vi "Teleop.vi"(10 "Match Info":T1={"Autonomous Elapsed Seconds"=0.0, "TeleOp Elapsed Seconds"=0.0, "Disabled Elapsed Seconds"=0.0, "Visited Autonomous"=FALSE, "Visited TeleOp"=FALSE, "Visited Disabled"=FALSE, "Autonomous Settings"={"Autonomous Style"=enum."Independent", "VI Refnum"=refnum}}, 11 "Call Context":T2) -> ()   [LabVIEW 2013]
doc: "This VI is called for each TeleOp packet received from the DS where the robot is not disabled. It is often used to read from the joysticks and update I/O or to update setpoints for timed control loops. It should complete and return within 20 milliseconds or it may miss DS packets."
uses:
  <vilib>/Rock Robotics/WPI/DriverStation/WPI_DriverStationDerivedRobotMode.ctl
  <vilib>/Rock Robotics/WPI/DriverStation/WPI_DriverStationMatch Info.ctl
  Robot Global Data.vi
  Gyro/Gyro Global.vi
  <vilib>/Rock Robotics/WPI/Joystick/WPI_JoystickGetSetRefNum.vi
panel:
  out "back":dbl
  out "front":dbl
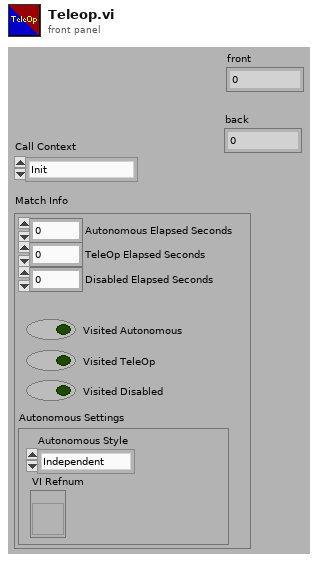
[diagram p1: front panel]
types:
  T1 = typedef "WPI_DriverStationMatch Info.ctl" = cluster{"Autonomous Elapsed Seconds":dbl, "TeleOp Elapsed Seconds":dbl, "Disabled Elapsed Seconds":dbl, "Visited Autonomous":bool, "Visited TeleOp":bool, "Visited Disabled":bool, "Autonomous Settings":cluster{"Autonomous Style":enum16{"Iterative", "Independent"}, "VI Refnum":refnum<vi>}}
  T2 = typedef "WPI_DriverStationDerivedRobotMode.ctl" = enum16{"Init", "Execute", "Stop"}
  T3 = typedef "WPI_JoystickDevRef.ctl" = cluster{"Device":T4}
  T4 = typedef "WPI_JoystickDeviceEnum.ctl" = enum16{"USB 1", "USB 2", "USB 3", "USB 4", "Kinect 1", "Kinect 2"}
  T5 = typedef "WPI_JoystickButtonState.ctl" = cluster{"Button 1":bool, "Button 2":bool, "Button 3":bool, "Button 4":bool, "Button 5":bool, "Button 6":bool, "Button 7":bool, "Button 8":bool, "Button 9":bool, "Button 10":bool, "Button 11":bool, "Button 12":bool}
  T6 = cluster{"axis 1 (x)":dbl, "axis 2 (y)":dbl, "axis 3 (throttle)":dbl, "axis 4":dbl, "axis 5":dbl, "axis 6":dbl}
  T7 = typedef "WPI_EncoderDevRef.ctl" = cluster{"DevStatus":errorcluster, "EncoderIndex":T8, "CounterIndex":T9, "DistancePerCount":dbl, "Decoding Type":T10}
  T8 = typedef "FPGA_EncoderIdx.ctl" = enum8{"Enc 0", "Enc 1", "Enc 2", "Enc 3", "Invalid"}
  T9 = typedef "FPGA_CounterCtrSystemIndex.ctl" = enum8{"Ctr 0", "Ctr 1", "Ctr 2", "Ctr 3", "Ctr 4", "Ctr 5", "Ctr 6", "Ctr 7", "Invalid"}
  T10 = typedef "WPI_EncoderType.ctl" = enum16{"1x", "2x", "4x"}
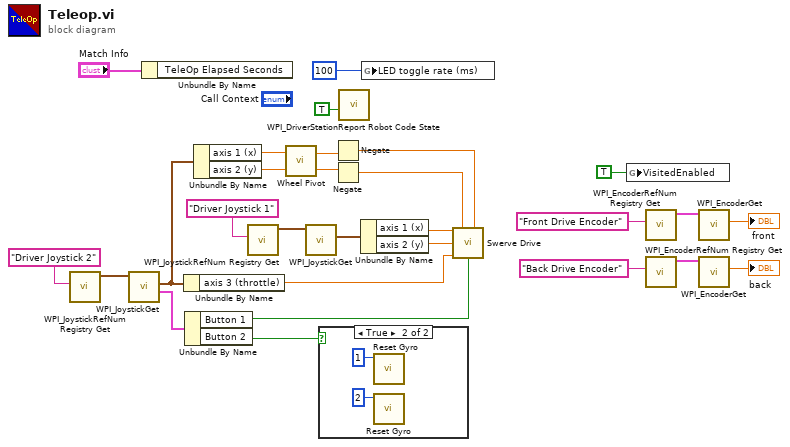
[diagram p0: block diagram]
diagram:
  n1 = call <vilib>:"WPI_JoystickRefNum Registry Get.vi"("refnum name"="Driver Joystick 2") -> ("JoystickDevRef"=w19:T3)  [unwired: 1 in, 9 out]
  n2 = call <vilib>:"WPI_JoystickGet.vi"("JoystickDevRef"=w19) -> ("Buttons"=w13:T5, "Axes"=w8:T6)  [unwired: 1 in, 4 out]
  n3 = Unbundle By Name("Match Info") -> ()  [unwired: 1 out]
  n4 = Unbundle By Name(w8) -> ("axis 3 (throttle)"=w11:dbl)
  n5 = Unbundle By Name(w13) -> ("Button 1"=w12:bool, "Button 2"=w25:bool)
  n6 = Unbundle By Name(w8) -> ("axis 1 (x)"=w18:dbl, "axis 2 (y)"=w17:dbl)
  n7 = call <vilib>:"WPI_JoystickRefNum Registry Get.vi"("refnum name"="Driver Joystick 1") -> ("JoystickDevRef"=w22:T3)  [unwired: 1 in, 9 out]
  n8 = call "Wheel Pivot.vi"("y in"=w17, "x in"=w18) -> ("y out"=w16:dbl, "x out"=w15:dbl)
  n9 = call <vilib>:"WPI_JoystickGet.vi"("JoystickDevRef"=w22) -> ("Axes"=w14:T6)  [unwired: 1 in, 5 out]
  n10 = case shown="True" w25 {
    frame False {
    }
    frame True {
      n11 = call "Reset Gyro.vi"("Gyro ID (1 or 2)"=1) -> ()  [unwired: 11 in]
      n12 = call "Reset Gyro.vi"("Gyro ID (1 or 2)"=2) -> ()  [unwired: 11 in]
    }
  }
  n13 = Negate(x=w15) -> (-x=w24:dbl)
  n14 = Negate(x=w16) -> (-x=w23:dbl)
  n15 = call <vilib>:"WPI_DriverStationReport Robot Code State.vi"("TeleOp"=TRUE ("Autonomous")) -> ()  [unwired: 10 in, 1 out]
  n16 = Unbundle By Name(w14) -> ("axis 1 (x)"=w10:dbl, "axis 2 (y)"=w9:dbl)
  n17 = global write "Robot Global Data.vi" "LED toggle rate (ms)"(u32 100 ("LED ms toggle rate")) -> ()
  n18 = call "Swerve Drive.vi"("X"=w10, "Rot. Point Y"=w23, "Rot. Point X"=w24, "Y"=w9, "Z"=w11, "Robot-Centric"=w12) -> ()  [unwired: 10 in]
  n19 = global write "Gyro Global.vi" "VisitedEnabled"(TRUE ("VisitedEnabled")) -> ()
  n20 = call <vilib>:"WPI_EncoderRefNum Registry Get.vi"("refnum name"="Front Drive Encoder") -> ("EncoderDevRef"=w6:T7)  [unwired: 9 in, 1 out]
  n21 = call <vilib>:"WPI_EncoderRefNum Registry Get.vi"("refnum name"="Back Drive Encoder") -> ("EncoderDevRef"=w3:T7)  [unwired: 9 in, 1 out]
  n22 = call <vilib>:"WPI_EncoderGet.vi"("EncoderDevRef"=w6) -> ("Distance"=→"front":dbl)  [unwired: 5 in, 5 out]
  n23 = call <vilib>:"WPI_EncoderGet.vi"("EncoderDevRef"=w3) -> ("Distance"=→"back":dbl)  [unwired: 5 in, 5 out]
